vi "NI-Linux-RT Shared Library Path (DNN).vi"() -> (0 "Path":path)   [LabVIEW 2020, in "common.lvlib"]
doc: "Obtain the path to the Shared Library on NI Linux RT"
uses:
  common.lvlib
  Library Name.ctl
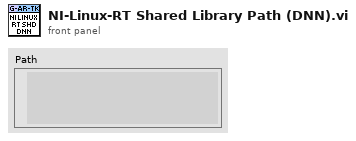
[diagram p1: front panel]
types:
  T1 = typedef "common.lvlib/Library Name.ctl" = enum16{"Core", "Feature Detection", "Augmented Reality", "DNN", "Tesseract", "Video IO"}
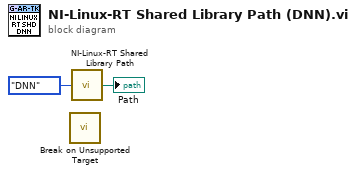
[diagram p0: block diagram]
diagram:
  n1 = call "Break on Unsupported Target.vi"() -> ()  [unwired: 12 in]
  n2 = call "NI-Linux-RT Shared Library Path.vi"("Library"=Library_Name."DNN") -> ("Path"=→"Path":path)
